vi "ni579x Validate Attenuation.vi"(0 "Register Bus":refnum<class "ni579x Register Bus v1 Host.lvclass">=refnum, 1 "scope":string, 5 "attenuation [dB]":dbl format="%#_6p", 11 "Error In":errorcluster) -> (4 "Register Bus (out)":refnum<class "ni579x Register Bus v1 Host.lvclass">, 6 "coerced attenuation [dB]":dbl format="%#_6p", 15 "Error Out":errorcluster)   [LabVIEW 2013]
uses:
  <instrlib>/ni579x/Register Bus/v1/Host/ni579x Register Bus v1 Host.lvclass
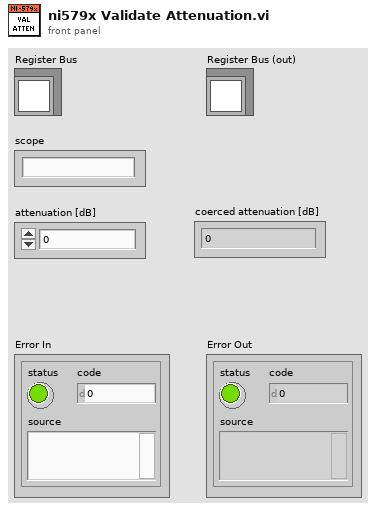
[diagram p1: front panel]
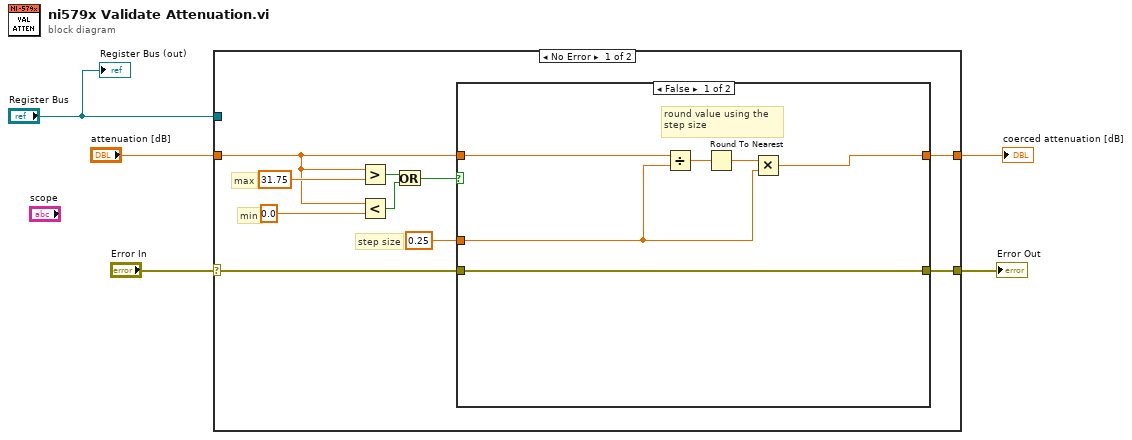
[diagram p0: block diagram]
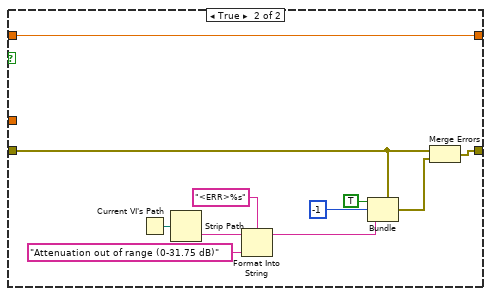
[diagram p2: hidden frame]
diagram:
  n1 = case shown="No Error" "Error In" {
    selector: "Error In" -> [w8 w34]
    tunnel: [w7 w34] -> w4
    tunnel: "Register Bus" -> [_ _]
    tunnel: "attenuation [dB]" -> [w10 w33]
    tunnel: [w6 w33] -> w1
    frame No Error {
      # "min"
      # "max"
      # "step size"
      n2 = Greater?(x=w10, y=31.75) -> (0:w13:bool)
      n3 = Less?(x=w10, y=0.0) -> (x < y?=w12:bool)
      n4 = Or(x=w13, y=w12) -> (x .or. y?=w11:bool)
      n5 = case shown="False" w11 {
        tunnel: w10 -> [w21 w25]
        tunnel: 0.25 -> [w17 _]
        tunnel: [w19 w25] -> w6
        tunnel: w8 -> [w18 w28]
        tunnel: [w18 w26] -> w7
        frame False {
          # "round value using the \nstep size"
          n6 = Divide(x=w21, y=w17) -> (x/y=w20:dbl)
          n7 = Round To Nearest(number=w20) -> (nearest integer value=w16:dbl)
          n8 = Multiply(x=w16, y=w17) -> (x*y=w19:dbl)
        }
        frame True {
          n9 = Current VI's Path() -> (path=w31:path)
          n10 = Strip Path(path=w31) -> (name=w30:string)  [unwired: 1 out]
          n11 = Format Into String(format string="<ERR>%s", initial string=w30, "Attenuation out of range (0-31.75 dB)" ("input 1")) -> (resulting string=w29:string)  [unwired: 1 in, 1 out]
          n12 = Bundle(cluster=w28, "status"=TRUE, "code"=-1, "source"=w29) -> (w27:errorcluster)
          n13 = Merge Errors(w28, w27) -> (w26:errorcluster)
        }
      }
    }
    frame Error {
    }
  }
  "Error Out" <- w4
  "coerced attenuation [dB]" <- w1
  "Register Bus (out)" <- "Register Bus"
